vi "Unscale and Scale - Grow Size.vi"(8 "error in (no error)":errorcluster, 11 "Data Scaling in":refnum<class "Data Scaling.lvclass">) -> (0 "error out":errorcluster, 3 "Data Scaling out":refnum<class "Data Scaling.lvclass">)   [LabVIEW 2020, in "Unit Tests.lvlib" / "Data Scaling.lvclass"]
uses:
  Data Scaling.lvclass
  Frames & Messages/TypeDefs/Scaling Information.ctl
  Frames & Messages/Utility/Scale Data.vi
  Frames & Messages/Utility/Unscale Data.vi
  <vilib>/addons/_JKI Toolkits/Caraya/classes/Assert/Assert True.vi
  <vilib>/addons/_JKI Toolkits/Caraya/classes/Test/Test.lvclass
  BCI-1553 API.lvlib
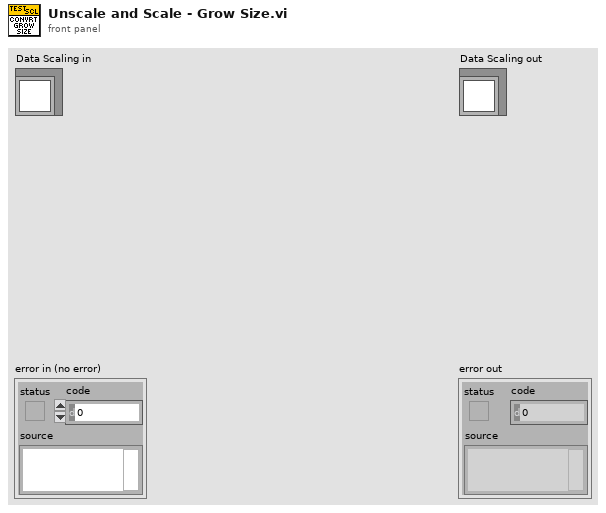
[diagram p1: front panel]
types:
  T1 = typedef "BCI-1553 API.lvlib/Scaling Information.ctl" = cluster{"Bit Offset":i32, "Bit Count":i32, "LSB Resolution":dbl, "2's Complement":bool, "Big Endian":bool, "Sign Bit":bool}
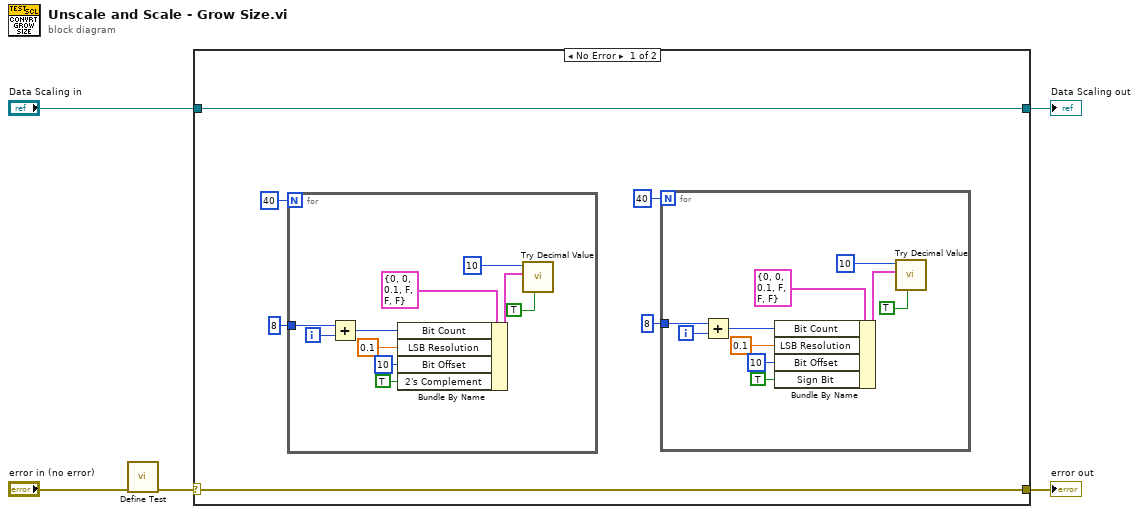
[diagram p0: block diagram]
diagram:
  n1 = call <vilib>:"Define Test.vi"("error in (no error)"="error in (no error)") -> ("error out"=w1:errorcluster)  [unwired: 9 in, 1 out]
  n2 = case shown="No Error" w1 {
    selector: w1 -> [w10 w33]
    tunnel: [w10 w33] -> w5
    tunnel: [w11 w32] -> w3
    tunnel: "Data Scaling in" -> [w11 w32]
    frame No Error {
      n3 = for {
        N: 40 -> [_]
        tunnel: 8 ("Bit Count") -> [w25]
        i -> [w23]
        n4 = Add(x=w25, y=w23) -> (x+y=w24:i32)
        n5 = Bundle By Name(cluster=T1 {"Bit Offset"=0, "Bit Count"=0, "LSB Resolution"=0.1, "2's Complement"=FALSE, "Big Endian"=FALSE, "Sign Bit"=FALSE} ("Scaling Info"), "Bit Count"=w24, "LSB Resolution"=0.1, "Bit Offset"=10, "2's Complement"=TRUE) -> (w28:T1)
        n6 = call "Try Decimal Value.vi"("Negate?"=TRUE, "Scaling Info"=w28, "Random Attempts"=10) -> ()  [unwired: 8 in, 1 out]
      }
      n7 = for {
        N: 40 -> [_]
        tunnel: 8 ("Bit Count") -> [w15]
        i -> [w13]
        n8 = Add(x=w15, y=w13) -> (x+y=w14:i32)
        n9 = Bundle By Name(cluster=T1 {"Bit Offset"=0, "Bit Count"=0, "LSB Resolution"=0.1, "2's Complement"=FALSE, "Big Endian"=FALSE, "Sign Bit"=FALSE} ("Scaling Info"), "Bit Count"=w14, "LSB Resolution"=0.1, "Bit Offset"=10, "Sign Bit"=TRUE) -> (w18:T1)
        n10 = call "Try Decimal Value.vi"("Negate?"=TRUE, "Scaling Info"=w18, "Random Attempts"=10) -> ()  [unwired: 8 in, 1 out]
      }
    }
    frame Error {
    }
  }
  "error out" <- w5
  "Data Scaling out" <- w3
